vi "_RT_CtrlLoop_Laser_Conv_Cmd.vi"(1 "Set Value":dbl format="%#_13g", 2 "Command Status":T1) -> (0 "Laser Command":string)   [LabVIEW 2018]
uses:
  Ctl/_ctl_LaserCmd.ctl
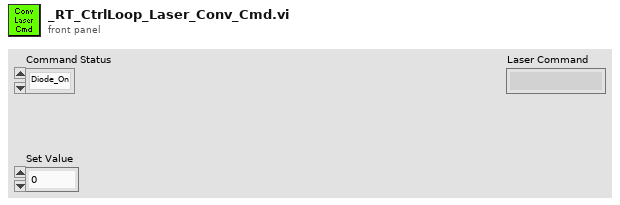
[diagram p1: front panel]
types:
  T1 = typedef "_ctl_LaserCmd.ctl" = enum8{"Diode_On", "Diode_Off", "Standby_On", "Standby_Off", "Internal_Trig", "External_Trig", "Set_Energy", "Set_Frequency", "Read_Version", "Read_STB", "Read_Diode_TEMP", "Read_SHG_TEMP", "Read_THG_TEMP", "Read_Base_Plate_TEMP", "Read_Diode_Hour", "Read_Diode_Maxc", "Read_Diode_Curr", "Read_QSW_CNTS", "Read_PENER", "Read_Freq", "Read_PCUR", "Read_Fault_Codes"}
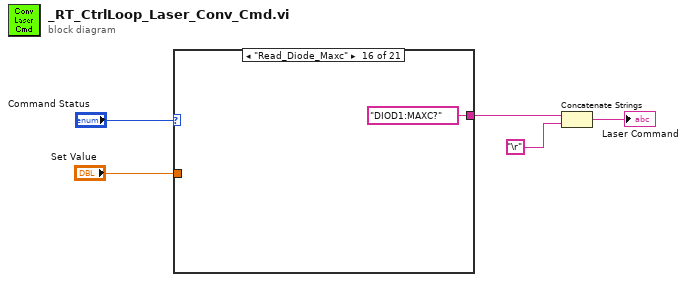
[diagram p0: block diagram]
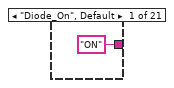
[diagram p2: hidden frame]
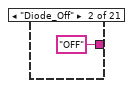
[diagram p3: hidden frame]
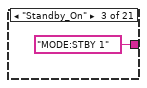
[diagram p4: hidden frame]
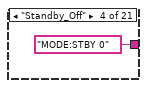
[diagram p5: hidden frame]
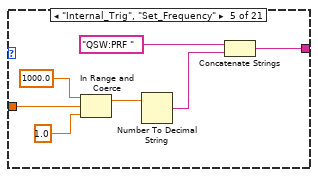
[diagram p6: hidden frame]
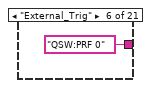
[diagram p7: hidden frame]
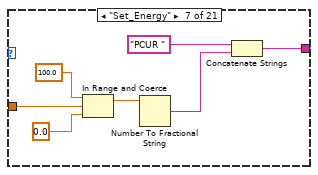
[diagram p8: hidden frame]
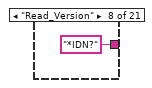
[diagram p9: hidden frame]
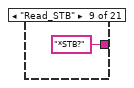
[diagram p10: hidden frame]
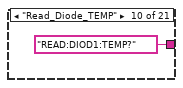
[diagram p11: hidden frame]
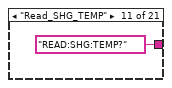
[diagram p12: hidden frame]
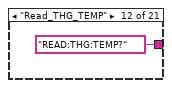
[diagram p13: hidden frame]
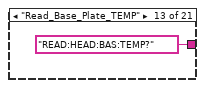
[diagram p14: hidden frame]
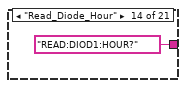
[diagram p15: hidden frame]
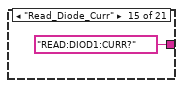
[diagram p16: hidden frame]
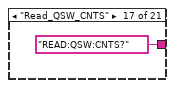
[diagram p17: hidden frame]
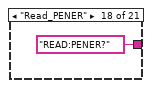
[diagram p18: hidden frame]
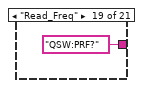
[diagram p19: hidden frame]
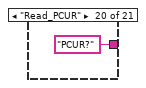
[diagram p20: hidden frame]
diagram:
  n1 = case shown="\"Read_Diode_Maxc\"" "Command Status" {
    tunnel: "Set Value" -> [_ _ _ _ w16 _ w20 _ _ _ _ _ _ _ _ _ _ _ _ _ _]
    tunnel: ["ON" "OFF" "MODE:STBY 1" "MODE:STBY 0" w11 "QSW:PRF 0" w18 "*IDN?" "*STB?" "READ:DIOD1:TEMP?" "READ:SHG:TEMP?" "READ:THG:TEMP?" "READ:HEAD:BAS:TEMP?" "READ:DIOD1:HOUR?" "READ:DIOD1:CURR?" "DIOD1:MAXC?" "READ:QSW:CNTS?" "READ:PENER?" "QSW:PRF?" "PCUR?" "READ:FAULT?"] -> w1
    frame "Diode_On", Default {
    }
    frame "Diode_Off" {
    }
    frame "Standby_On" {
    }
    frame "Standby_Off" {
    }
    frame "Internal_Trig", "Set_Frequency" {
      n2 = In Range and Coerce(upper limit=1000.0, x=w16, lower limit=1.0) -> (coerced(x)=w13:dbl)  [unwired: 1 out]
      n3 = Number To Decimal String(number=w13) -> (decimal integer string=w10:string)  [unwired: 1 in]
      n4 = Concatenate Strings("QSW:PRF ", w10) -> (w11:string)
    }
    frame "External_Trig" {
    }
    frame "Set_Energy" {
      n5 = In Range and Coerce(upper limit=100.0, x=w20, lower limit=0.0) -> (coerced(x)=w22:dbl)  [unwired: 1 out]
      n6 = Number To Fractional String(number=w22) -> (F-format string=w21:string)  [unwired: 3 in]
      n7 = Concatenate Strings("PCUR " ("string to write"), w21) -> (w18:string)
    }
    frame "Read_Version" {
    }
    frame "Read_STB" {
    }
    frame "Read_Diode_TEMP" {
    }
    frame "Read_SHG_TEMP" {
    }
    frame "Read_THG_TEMP" {
    }
    frame "Read_Base_Plate_TEMP" {
    }
    frame "Read_Diode_Hour" {
    }
    frame "Read_Diode_Curr" {
    }
    frame "Read_Diode_Maxc" {
    }
    frame "Read_QSW_CNTS" {
    }
    frame "Read_PENER" {
    }
    frame "Read_Freq" {
    }
    frame "Read_PCUR" {
    }
    frame "Read_Fault_Codes" {
    }
  }
  n8 = Concatenate Strings(w1, "\r") -> (→"Laser Command":string)
